vi "SaveProcData.vi"(9 "File Paths":T1={"Local Save Path"=path "\\\\smbhome.uscs.susx.ac.uk\\cv222/Desktop/data", "Newton Save Path"=path "Z:/#Projects/Entanglement/data", "File Name"="test", "LocalSave"=TRUE}, 10 "probs list":dbl[](array[numeric]), 11 "params in":string) -> ()   [LabVIEW 2019]
uses:
  controls/FilePaths.ctl
  controls/GlobalExp.vi
  <vilib>/Utility/file.llb/Write To Spreadsheet File (string).vi
  Global.lvlib
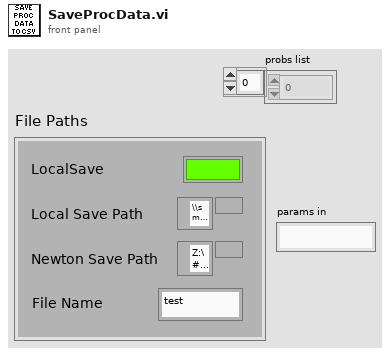
[diagram p1: front panel]
types:
  T1 = typedef "FilePaths.ctl" = cluster{"Local Save Path":path, "Newton Save Path":path, "File Name":string, "LocalSave":bool}
  T2 = typedef "MasterExpControl.ctl" = cluster{"Main Steps":dbl, "Main Runs":dbl, "ExpStatus":enum16{"Innit", "Stop", "Idle", "MainRunning", "AuxRunning"}, "Main Current Step":dbl, "ExpNum":dbl, "NewData":bool, "date":string, "command":string, "Stop":bool, "Pause":bool, "Mathematica":string, "Main/Meta":bool, "UpdateMath":bool, "Camera":bool, "MetaExpOver":bool, "NextMetaExp":bool}
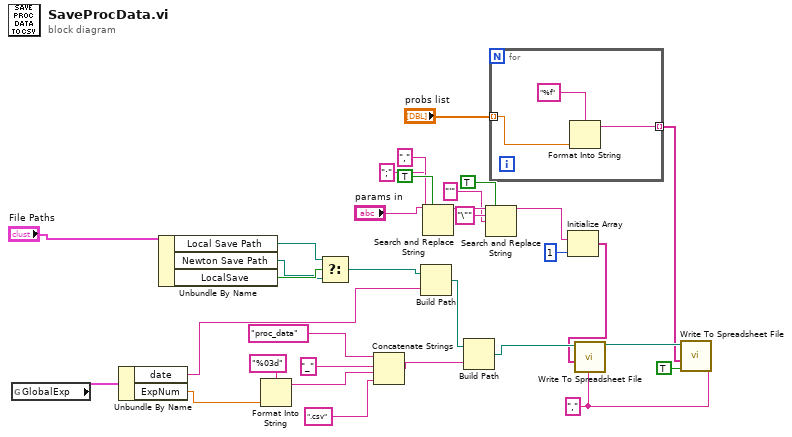
[diagram p0: block diagram]
diagram:
  w11 = "," ("delimiter (\\t)")
  n1 = global read "GlobalExp.vi" "GlobalExp"() -> (w29:T2)
  n2 = Unbundle By Name(w29) -> ("date"=w22:string, "ExpNum"=w20:dbl)
  n3 = Unbundle By Name("File Paths") -> ("Local Save Path"=w30:path, "Newton Save Path"=w31:path, "LocalSave"=w32:bool)
  n4 = Format Into String(format string="%03d", w20) -> (resulting string=w25:string)  [unwired: 2 in, 1 out]
  n5 = Select(t=w30, s=w32, f=w31) -> (s? t:f=w23:path)
  n6 = Concatenate Strings("proc_data" ("string"), "_", w25, ".csv") -> (w27:string)
  n7 = Build Path(base path=w23, name or relative path=w22) -> (appended path=w21:path)
  n8 = Search and Replace String(replace all?=TRUE ("replace all? (F)"), input string="params in", search string=",", replace string=";" ("replace string (\"\")")) -> (result string=w3:string)  [unwired: 4 in, 3 out]
  n9 = Build Path(base path=w21, name or relative path=w27) -> (appended path=w17:path)
  n10 = Search and Replace String(replace all?=TRUE ("replace all? (F)"), input string=w3, search string="\"", replace string="'" ("replace string (\"\")")) -> (result string=w5:string)  [unwired: 4 in, 3 out]
  n11 = for {
    tunnel: "probs list" -> [w34] mode=indexing
    tunnel: [w33] -> w12 mode=indexing
    n12 = Format Into String(format string="%f", w34) -> (resulting string=w33:string)  [unwired: 2 in, 1 out]
  }
  n13 = Initialize Array(w5, 1 ("dimension size")) -> (w15:string[])
  n14 = call-poly <vilib>:"Write To Spreadsheet File.vi"("delimiter (\\t)"=w11, "1D data"=w15, "file path (dialog if empty)"=w17) -> ("new file path (Not A Path if cancelled)"=w13:path)  [unwired: 5 in]
  n15 = call-poly <vilib>:"Write To Spreadsheet File.vi"("delimiter (\\t)"=w11, "append to file? (new file:F)"=TRUE, "1D data"=w12, "file path (dialog if empty)"=w13) -> ()  [unwired: 4 in, 1 out]
